vi "Read Default Value.vi"(8 "error in (no error)":errorcluster, 11 "List Data Type in":refnum<class "List Data Type.lvclass">) -> (0 "error out":errorcluster, 2 "Default Value":string, 3 "List Data Type out":refnum<class "List Data Type.lvclass">)   [LabVIEW 2018, in "List Data Type.lvclass"]
uses:
  List Data Type.lvclass
  List Data Type.lvclass/List Data Type.ctl
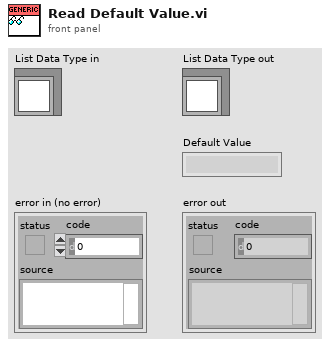
[diagram p1: front panel]
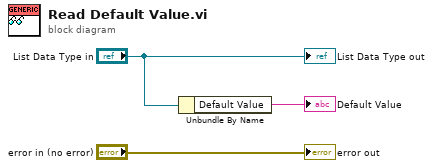
[diagram p0: block diagram]
diagram:
  n1 = Unbundle By Name("List Data Type in") -> ("Default Value"=→"Default Value":string)
  "error out" <- "error in (no error)"
  "List Data Type out" <- "List Data Type in"
